vi "RSI Module_UI.vi"(8 "error in (no error)":errorcluster, 11 "Node Ptr":T3 format="%.0x") -> (0 "error out":errorcluster)   [LabVIEW 2011, in "Modules.lvlib" / "RSI Module.lvclass"]
uses:
  RSI Module.lvclass
  <vilib>/NI Veristand/Custom Device API/Custom Device Item Ref.ctl
  SubPanel Command.ctl
  Channels.ctl
  Channel Type.ctl
  <vilib>/NI Veristand/Custom Device API/Custom Device API.lvlib
panel:
  out "Channels":T1
  in  "SubPanel Event":refnum<user-event>
  in  "Header":cluster{"Section Name":string}={"Section Name"="Custom Device Item Settings"}
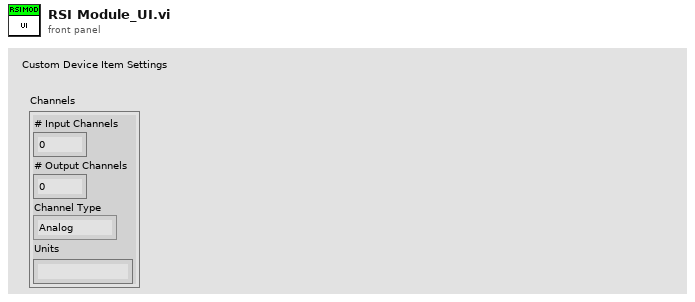
[diagram p1: front panel]
types:
  T1 = typedef "Modules.lvlib/RSI Module.lvclass/Channels.ctl" = cluster{"# Input Channels":i32, "# Output Channels":i32, "Channel Type":T2, "Units":string}
  T2 = typedef "Modules.lvlib/RSI Module.lvclass/Channel Type.ctl" = enum16{"Analog", "Digital"}
  T3 = typedef "Custom Device API.lvlib/Custom Device Item Ref.ctl" = u64
  T4 = typedef "Modules.lvlib/RSI Module.lvclass/SubPanel Command.ctl" = enum16{"Stop"}
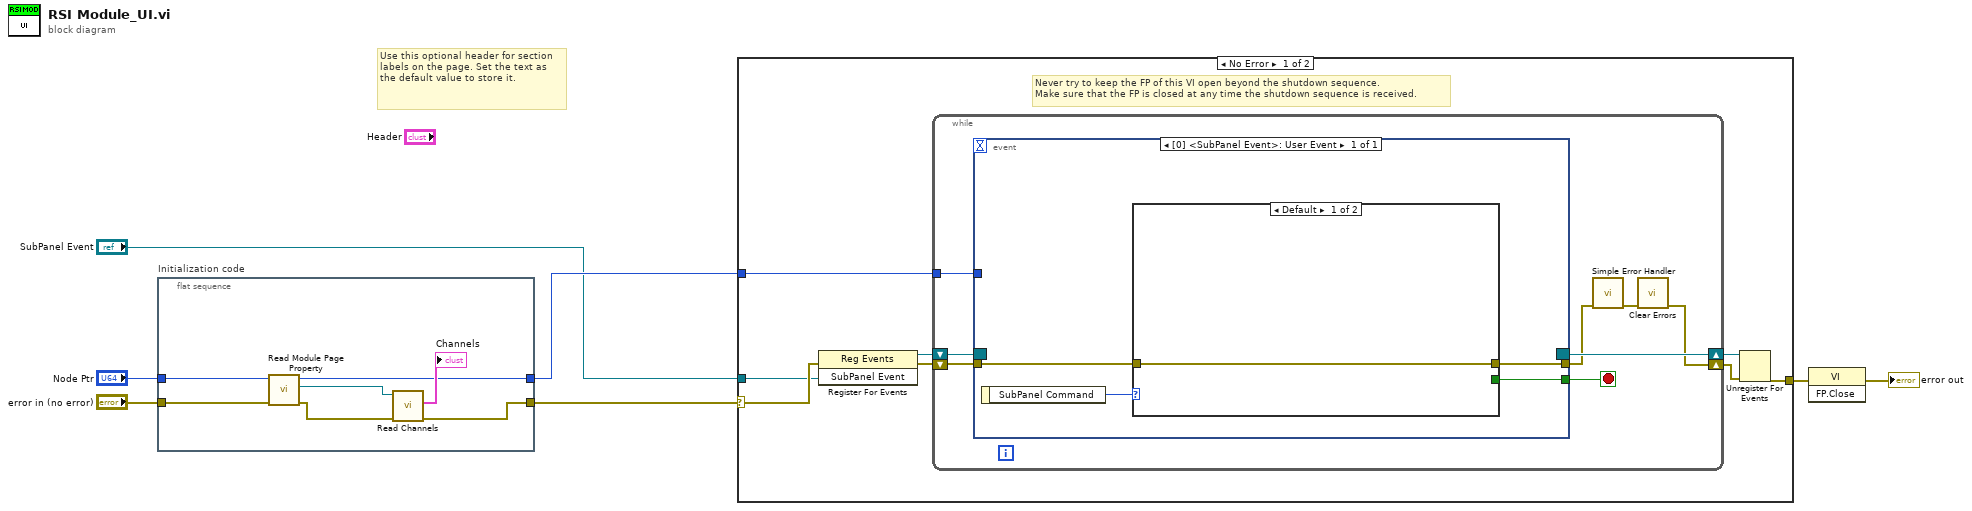
[diagram p0: block diagram]
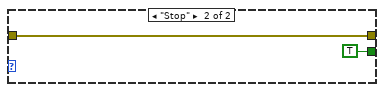
[diagram p2: hidden frame]
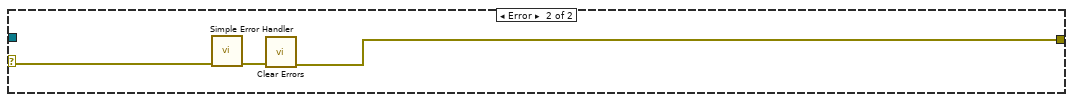
[diagram p3: hidden frame]
diagram:
  # "Use this optional header for section labels on the page. Set the text as the default value to store it."
  n1 = flat-sequence "Initialization code" {
    tunnel: "error in (no error)" -> [w11]
    tunnel: "Node Ptr" -> [w12]
    tunnel: [w14] -> w1
    tunnel: [w10] -> w4
    frame #0 {
      n2 = call "Read Module Page Property.vi"("error in (no error)"=w11, "Node Ptr In"=w12) -> ("error out"=w8:errorcluster, "RSI Module"=w9:refnum<class "RSI Module.lvclass">, "Node Ptr Out"=w10:T3)  [unwired: 7 in]
      n3 = call "Read Channels.vi"("error in (no error)"=w8, "RSI Module in"=w9) -> ("error out"=w14:errorcluster, "Channels"=→"Channels":T1)  [unwired: 7 in, 1 out]
    }
  }
  n4 = case shown="No Error" w1 {
    selector: w1 -> [w16 w40]
    tunnel: [w20 w38] -> w7
    tunnel: w4 -> [w17 _]
    tunnel: "SubPanel Event" -> [w15 _]
    frame No Error {
      # "Never try to keep the FP of this VI open beyond the shutdown sequence.\nMake sure that the FP is closed at any time the shutdown sequence is received."
      n5 = register-events(error in=w16, w15) -> (reference out=w18:refnum<event-registration>, error out=w19:errorcluster)  [unwired: 1 in]
      n6 = while {
        tunnel: w17 -> [w26]
        shift-right: [w23] -> w21
        shift-left: w19 -> [w29]
        shift-right: [w30] -> w22
        shift-left: w18 -> [w28]
        stop <- w27 stop-if-true
        n7 = event shown="[0] <SubPanel Event>: User Event" {
          selector: w28 -> [_]
          dyn-events: [_] -> w30
          timeout: _ -> [_]
          tunnel: w29 -> [w33]
          tunnel: [w31] -> w27
          tunnel: [w32] -> w25
          tunnel: w26 -> [_]
          event User Event {
            n8 = event-data() -> ("SubPanel Command"=w34:T4)  [unwired: 1 out]
            n9 = case shown="Default" w34 {
              tunnel: w33 -> [w35 w36]
              tunnel: [w35 w36] -> w32
              tunnel: [_ TRUE] -> w31
              frame Default {
              }
              frame "Stop" {
              }
            }
          }
        }
        n10 = call <vilib>:"Simple Error Handler.vi"("error in (no error)"=w25) -> ("error out"=w24:errorcluster)  [unwired: 1 in, 7 out]
        n11 = call <vilib>:"Clear Errors.vi"("error in (no error)"=w24) -> ("error out"=w23:errorcluster)  [unwired: 6 out]
      }
      n12 = Unregister For Events(event registration refnum=w22, error in=w21) -> (error out=w20:errorcluster)
    }
    frame Error {
      n13 = call <vilib>:"Simple Error Handler.vi"("error in (no error)"=w40) -> ("error out"=w39:errorcluster)  [unwired: 1 in, 7 out]
      n14 = call <vilib>:"Clear Errors.vi"("error in (no error)"=w39) -> ("error out"=w38:errorcluster)  [unwired: 6 out]
    }
  }
  n15 = invoke class="VI" method="FP.Close"(error in=w7) -> (error out=→"error out":errorcluster)  [unwired: 2 in, 2 out]
